vi "Data Cluster to Feedback Array.vi"(3 "InstDataCluster":T1) -> (1 "Inst FB":dbl[](array[numeric]))   [LabVIEW 2013]
uses:
  TypeDef/DataCluster.ctl
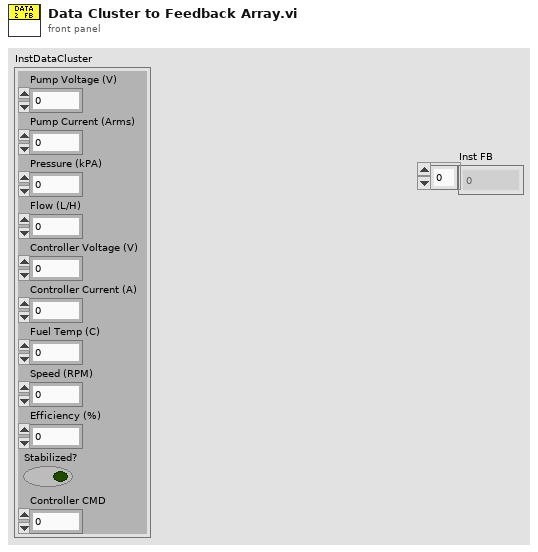
[diagram p1: front panel]
types:
  T1 = typedef "DataCluster.ctl" = cluster{"Pump Voltage (V)":dbl, "Pump Current (Arms)":dbl, "Pressure (kPA)":dbl, "Flow (L/H)":dbl, "Controller Voltage (V)":dbl, "Controller Current (A)":dbl, "Fuel Temp (C)":dbl, "Speed (RPM)":dbl, "Efficiency (%)":dbl, "Stabilized?":bool, "Controller CMD":dbl}
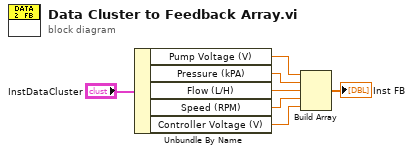
[diagram p0: block diagram]
diagram:
  n1 = Unbundle By Name("InstDataCluster") -> ("Pump Voltage (V)"=w6:dbl, "Pressure (kPA)"=w5:dbl, "Flow (L/H)"=w4:dbl, "Speed (RPM)"=w3:dbl, "Controller Voltage (V)"=w2:dbl)
  n2 = Build Array(w6, w5, w4, w3, w2) -> (→"Inst FB":dbl[])
